vi "GetIntFromNode(viaStringNodePath).vi"(2 "Path":string, 3 "error in":errorcluster, 5 "Tree DVR in":refnum<data-value>) -> (0 "error out":errorcluster, 1 "Int32":i32)   [LabVIEW 2013]
uses:
  <vilib>/MDSplus/Classes/Tree_Class/Tree.lvclass
  <vilib>/MDSplus/Library/MDSplus.lvlib
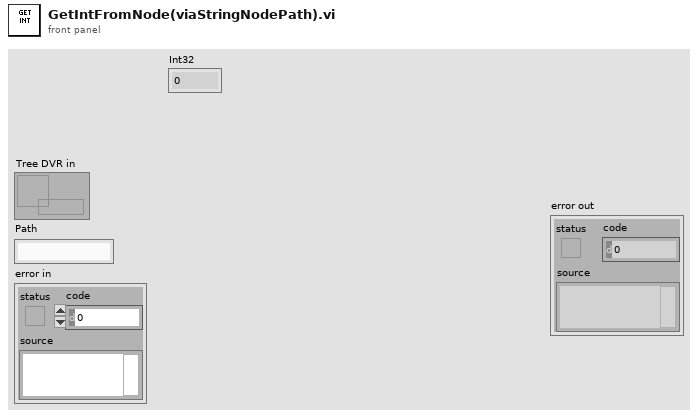
[diagram p1: front panel]
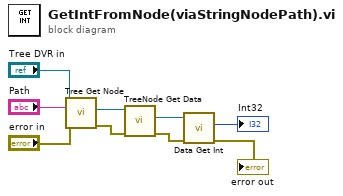
[diagram p0: block diagram]
diagram:
  n1 = call <vilib>:"Tree Get Node.vi"("error in (no error)"="error in", "Path"="Path", "Tree DVR in"="Tree DVR in") -> ("error out"=w8:errorcluster, "Node out"=w9:refnum<data-value>)  [unwired: 6 in, 1 out]
  n2 = call <vilib>:"TreeNode Get Data.vi"("error in (no error)"=w8, "TreeNode DVR in"=w9) -> ("error out"=w7:errorcluster, "Data out"=w6:refnum<data-value>)  [unwired: 7 in, 1 out]
  n3 = call <vilib>:"Data Get Int.vi"("error in (no error)"=w7, "Data DVR in"=w6) -> ("error out"=→"error out":errorcluster, "I32 out"=→"Int32":i32)  [unwired: 7 in, 1 out]
